vi "T14 - Тестирование Lister.vi"() -> ()   [LabVIEW 2009]
uses:
  Z210/Z210 CTL Lib.llb/Z210 CTL ADC or DAC Function.ctl
  Z210/Z210 CTL Lib.llb/Z210 CTL ADC Linear Correction.ctl
panel:
  in  "Число измерений":i32=5
  in  "Номер канала DAC":i32
  in  "Опросить пользователя с клавиатуры?":bool=TRUE
  out "ADC Voltages":dbl[unit][][](array[numeric])
  in  "Linear Correction ADC":T1=[{"scale"=1.0, "offset"=0.0}, {"scale"=1.0, "offset"=0.0}, {"scale"=1.0, "offset"=0.0}, {"scale"=1.0, "offset"=0.0}, {"scale"=1.0, "offset"=0.0}, {"scale"=1.0, "offset"=0.0}, {"scale"=1.0, "offset"=0.0}, {"scale"=1.0, "offset"=0.0}, {"scale"=1.0, "offset"=0.0}, {"scale"=1.0, "offset"=0.0}, {"scale"=1.0, "offset"=0.0}, {"scale"=1.0, "offset"=0.0}, {"scale"=1.0, "offset"=0.0}, {"scale"=1.0, "offset"=0.0}, {"scale"=1.0, "offset"=0.0}, {"scale"=1.0, "offset"=0.0}]
  # "Это отладка для subVI используемого для калибровки. Измерение в данном случае следующее на указанном канале ЦАП устанавливается напряжение в диапазоне 0 - 2,5В (на другом канале ЦАП 0 вольт)\nЗатем записываются показания всех каналов АЦП и, если было указано, опрашивается пользователь. Введенное пользователем записывается отдельным каналом в конец."
  # "0. Для этого теста потребуется внешний вольтметр.\n1. Соединить:\n    • DAC#0 <-> ADC#0\n    • DAC#1 <-> ADC#1\n2. Указать номер канала (0 либо 1), число измерений (5 вполне достаточно) и\nопросить пользователя = true. Остальное по желанию.\n3. Подключить вольтметр параллельно к выбранному каналу.\n3. Запустить. Следовать инструкциям на вспывающих окнах.\n4. Смотреть структуру вывода ADC Voltages"
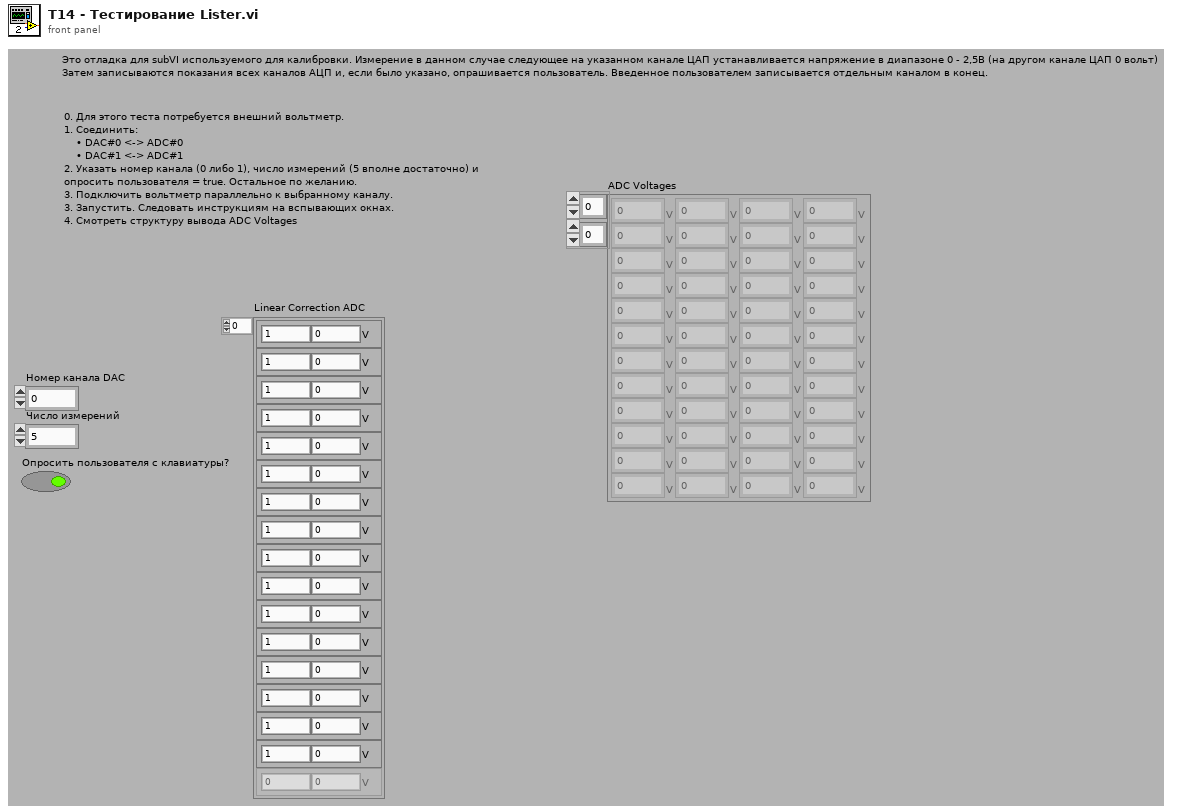
[diagram p1: front panel]
types:
  T1 = typedef "Z210 CTL ADC Linear Correction.ctl" = cluster{"scale":dbl, "offset":dbl[unit]}[]
  T2 = typedef "Z210 CTL ADC or DAC Function.ctl" = enum16{"АЦП", "ЦАП", "Both"}
  T3 = typedef "Z210 CTL Unit Data .ctl" = cluster{"typeDevice":i32, "numberDSP":i32}
  T4 = typedef "Z210 CTL Buffers Params.ctl" = cluster{"bufferAddr ADC":u32, "bufferSize ADC":i32, "bufferAddr DAC":u32, "bufferSize DAC":i32}
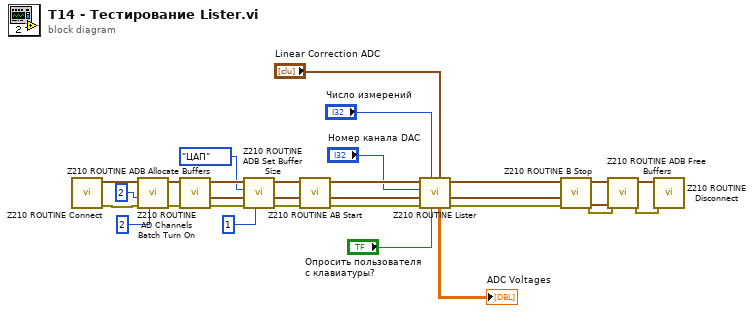
[diagram p0: block diagram]
diagram:
  n1 = call "Z210 ROUTINE Connect.vi"() -> ("error out"=w29:errorcluster, "unitData out"=w30:T3)  [unwired: 10 in]
  n2 = call "Z210 ROUTINE AD Channels Batch Turn On.vi"("N ЦАП (0)"=2, "error in (no error)"=w29, "N Синф (0)"=2, "unitData in"=w30) -> ("error out"=w27:errorcluster, "unitData out"=w28:T3)  [unwired: 4 in, 2 out]
  n3 = call "Z210 ROUTINE ADB Allocate Buffers.vi"("error in (no error)"=w27, "unitData in"=w28) -> ("error out"=w21:errorcluster, "buffersParams out"=w24:T4, "unitData out"=w23:T3)  [unwired: 7 in]
  n4 = call "Z210 ROUTINE ADB Set Buffer Size.vi"("size suggestion (0)"=1, "error in (no error)"=w21, "buffersParams"=w24, "AorD"=Z210_CTL_ADC_or_DAC_Function."ЦАП", "unitData in"=w23) -> ("error out"=w18:errorcluster, "buffersParams out"=w17:T4, "unitData out"=w19:T3)  [unwired: 4 in]
  n5 = call "Z210 ROUTINE AB Start.vi"("error in (no error)"=w18, "buffersParams"=w17, "unitData in"=w19) -> ("error out"=w9:errorcluster, "buffersParams out"=w10:T4, "unitData out"=w11:T3)  [unwired: 6 in]
  n6 = call "Z210 ROUTINE Lister.vi"("Linear Correction ADC"="Linear Correction ADC", "PromptUser?"="Опросить пользователя с клавиатуры?", "Points"="Число измерений", "error in (no error)"=w9, "buffersParams"=w10, "DAC#"="Номер канала DAC", "unitData in"=w11) -> ("error out"=w5:errorcluster, "buffersParams out"=w6:T4, "unitData out"=w8:T3, "Array"=→"ADC Voltages":dbl[unit][][])  [unwired: 1 in]
  n7 = call "Z210 ROUTINE B Stop.vi"("error in (no error)"=w5, "buffersParams"=w6, "unitData in"=w8) -> ("error out"=w14:errorcluster, "buffersParams out"=w15:T4, "unitData out"=w16:T3)  [unwired: 6 in]
  n8 = call "Z210 ROUTINE ADB Free Buffers.vi"("error in (no error)"=w14, "buffersParams"=w15, "unitData in"=w16) -> ("error out"=w12:errorcluster, "unitData out"=w13:T3)  [unwired: 6 in, 1 out]
  n9 = call "Z210 ROUTINE Disconnect.vi"("error in (no error)"=w12, "unitData in"=w13) -> ()  [unwired: 8 in, 2 out]
